vi "ADCP_get_all_parameters.vi"(8 "error in (no error)":errorcluster, 11 "ADCP In":refnum<class "ADCP.lvclass">) -> (0 "error out":errorcluster, 1 "Parameter names":string[](array[string]), 2 "Parameters":T1(array[cluster]), 3 "ADCP Out":refnum<class "ADCP.lvclass">)   [LabVIEW 2017, in "ADCP.lvclass"]
uses:
  ADCP.lvclass
  ADCP.lvclass/ADCP.ctl
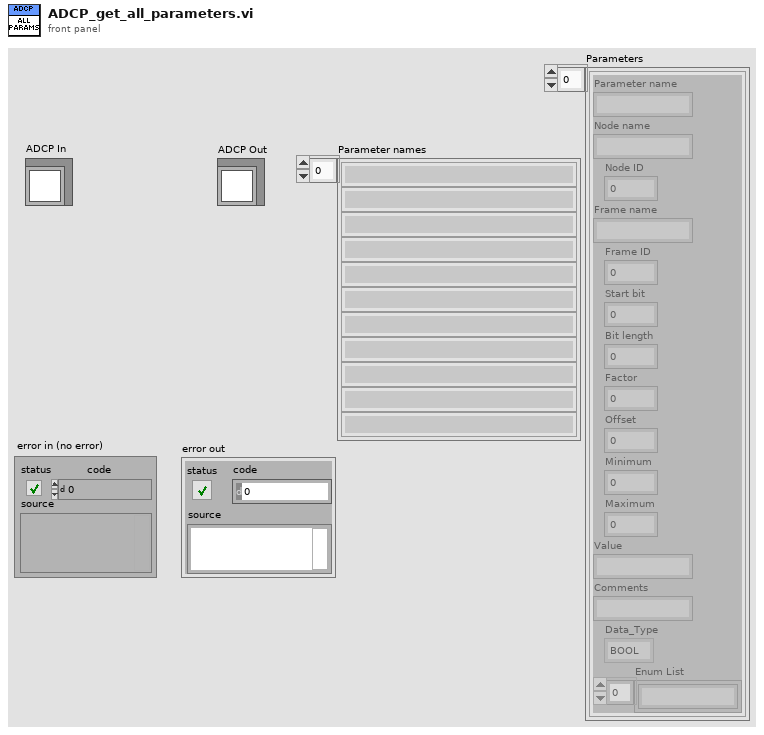
[diagram p1: front panel]
types:
  T1 = cluster{"Parameter name":string, "Node name":string, "Node ID":u8, "Frame name":string, "Frame ID":u8, "Start bit":u32, "Bit length":u32, "Factor":dbl, "Offset":dbl, "Minimum":dbl, "Maximum":dbl, "Value":string, "Comments":string, "Data_Type":enum16{"BOOL", "UNSIGNED", "SIGNED", "FLOAT32", "ENUM"}, "Enum List":string[]}[]
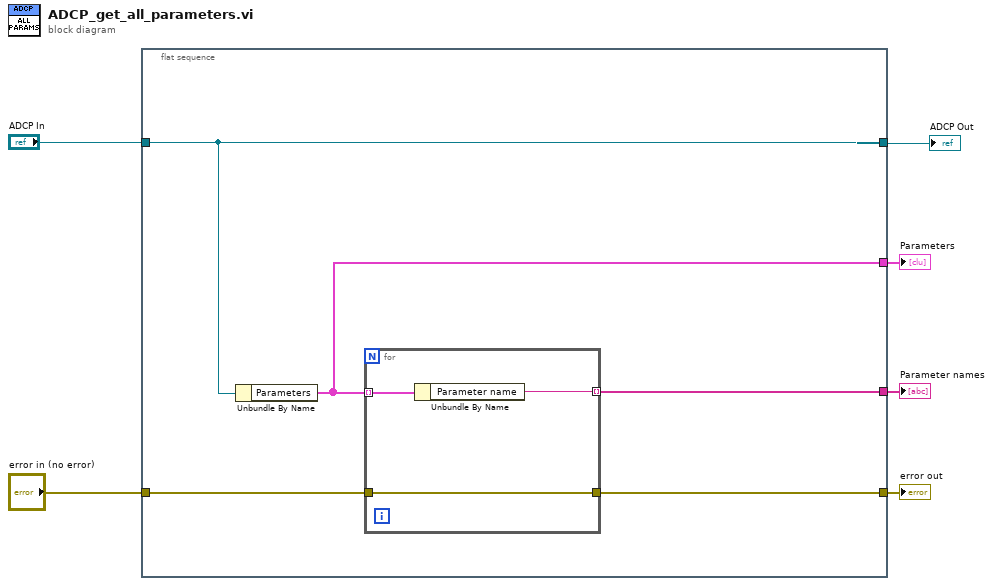
[diagram p0: block diagram]
diagram:
  n1 = flat-sequence {
    tunnel: "ADCP In" -> [w11]
    tunnel: [w11] -> w5
    tunnel: "error in (no error)" -> [w10]
    tunnel: [w9] -> w1
    tunnel: [w8] -> w2
    tunnel: [w7] -> w3
    frame #0 {
      n2 = Unbundle By Name(w11) -> ("Parameters"=w7:T1)
      n3 = for {
        tunnel: w10 -> [w14]
        tunnel: [w14] -> w9
        tunnel: w7 -> [w13] mode=indexing
        tunnel: [w12] -> w8 mode=indexing
        n4 = Unbundle By Name(w13) -> ("Parameter name"=w12:string)
      }
    }
  }
  "ADCP Out" <- w5
  "Parameters" <- w3
  "Parameter names" <- w2
  "error out" <- w1
